vi "Matches.vi"(8 "error in (no error)":errorcluster, 10 "Actual":variant, 11 "IsRefnum in":refnum<class "IsRefnum.lvclass">) -> (0 "error out":errorcluster, 2 "Result":bool, 3 "IsRefnum out":refnum<class "IsRefnum.lvclass">)   [LabVIEW 2019, in "Constraint.lvlib" / "IsRefnum.lvclass"]
doc: "Evaluates the constraint for <B>Actual</B>. Returns true if the constraint is met."
uses:
  IsRefnum.lvclass
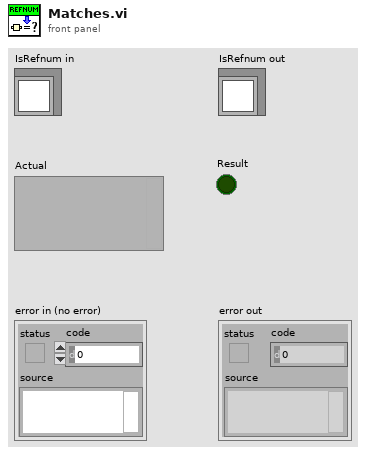
[diagram p1: front panel]
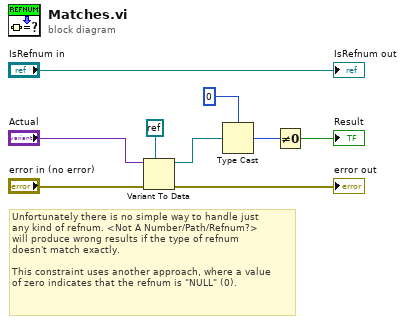
[diagram p0: block diagram]
diagram:
  # "Unfortunately there is no simple way to handle just\nany kind of refnum. <Not A Number/Path/Refnum?>\nwill produce wrong results if the type of refnum\ndoesn't match exactly.\n\nThis constraint uses another approach, where a value\nof zero indicates that the refnum is \"NULL\" (0)."
  n1 = Variant To Data(error in="error in (no error)", type=refnum<k0> refnum, Variant="Actual") -> (data=w6:refnum<k0>, error out=→"error out":errorcluster)
  n2 = Type Cast(type=i64 0, x=w6) -> (*(type *) &x=w3:i64)
  n3 = Not Equal To 0?(x=w3) -> (x != 0?=→"Result":bool)
  "IsRefnum out" <- "IsRefnum in"
